vi "Begin.vi"(8 "error in":errorcluster) -> (0 "error out":errorcluster)   [LabVIEW 2017]
doc: "Called before other user functions, this VI is expected to open initial I/O refnums, load in file data, and do all program initialization. Notice that the <B>error out</B> terminal is simply used for data flow. Wiring it to other structures or subVIs ensures that this VI runs first."
uses:
  <vilib>/Rock Robotics/WPI/DriverStation/WPI_DriverStationRobotMode2.ctl
  <vilib>/Rock Robotics/WPI/Joystick/WPI_JoystickDeviceEnum.ctl
  <vilib>/Rock Robotics/SystemInterfaces/DIO/FPGA_DIOPWMChannel.ctl
  <vilib>/Rock Robotics/WPI/SafetyOutput/WPI_SafetyOutputConfigMenu.ctl
  Robot Global Data.vi
  <vilib>/Rock Robotics/Network Tables/NT Write String Array.vi
  <vilib>/Rock Robotics/WPI/MotorControl/WPI_MotorControlOpen VictorSP.vi
  <vilib>/Rock Robotics/WPI/MotorControl/WPI_MotorControlOpen SPARK.vi
  <vilib>/Rock Robotics/WPI/RobotDrive/WPI_RobotDriveOpen4MotorWithExistingMotors.vi
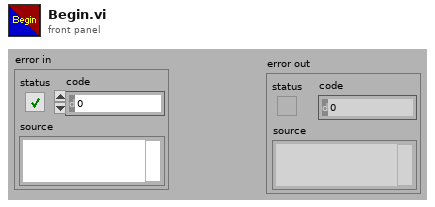
[diagram p1: front panel]
types:
  T1 = typedef "WPI_SafetyOutputConfigMenu.ctl" = enum16{"Enable", "Disable"}
  T2 = typedef "FPGA_DIOPWMChannel.ctl" = enum8{"PWM 0", "PWM 1", "PWM 2", "PWM 3", "PWM 4", "PWM 5", "PWM 6", "PWM 7", "PWM 8", "PWM 9", "PWM MXP 0", "PWM MXP 1", "PWM MXP 2", "PWM MXP 3", "PWM MXP 4", "PWM MXP 5", "PWM MXP 6", "PWM MXP 7", "PWM MXP 8", "PWM MXP 9", "Invalid"}
  T3 = typedef "WPI_JoystickDeviceEnum.ctl" = enum16{"USB 0", "USB 1", "USB 2", "USB 3", "USB 4", "USB 5"}
  T4 = typedef "WPI_DriverStationRobotMode2.ctl" = enum16{"Autonomous Disabled", "Autonomous Enabled", "Teleop Disabled", "Teleop Enabled", "Disconnected", "Finish", "Test Disabled", "Test Enabled", "Emergency Stopped"}
  T5 = typedef "WPI_JoystickDevRef.ctl" = cluster{"Device":T3}
  T6 = typedef "WPI_MotorControlDeviceRef.ctl" = cluster{"DeviceStatus":errorcluster, "Type":T7, "PWM":cluster{"PWM Channel":T2, "DeadBand":T8}, "CAN":cluster{"Device Number":u8, "SetOutput VI Ref":variant, "GetOutput VI Ref":variant, "Enable VI Ref":variant, "Disable VI Ref":variant, "Data":variant}, "Invert":bool, "DIO PWM":cluster{"PWM \"Enable\" Channel":T2, "DIOChannel":T9, "PWM Rate":dbl}}
  T7 = typedef "WPI_MotorControlType.ctl" = enum16{"PWM", "CAN", "DIO PWM"}
  T8 = typedef "WPI_PWMDeadband.ctl" = cluster{"Name":string, "maxPositivePwm":i32, "minPositivePwm":i32, "centerPwm":i32, "maxNegativePwm":i32, "minNegativePwm":i32, "angularRange":u16}
  T9 = typedef "FPGA_DIOChannel.ctl" = enum8{"DIO 0", "DIO 1", "DIO 2", "DIO 3", "DIO 4", "DIO 5", "DIO 6", "DIO 7", "DIO 8", "DIO 9", "DIO MXP 0", "DIO MXP 1", "DIO MXP 2", "DIO MXP 3", "DIO MXP 4", "DIO MXP 5", "DIO MXP 6", "DIO MXP 7", "DIO MXP 8", "DIO MXP 9", "DIO MXP 10", "DIO MXP 11", "DIO MXP 12", "DIO MXP 13", "DIO MXP 14", "DIO MXP 15", "SPI Port CS1", "SPI Port CS2", "SPI Port CS3", "SPI Port MISO", "SPI Port MOSI", "Invalid"}
  T10 = typedef "WPI_RobotDriveDevRef.ctl" = cluster{"DevStatus":errorcluster, "Motors[]":T6[], "Square Inputs":bool, "Max Output":dbl}
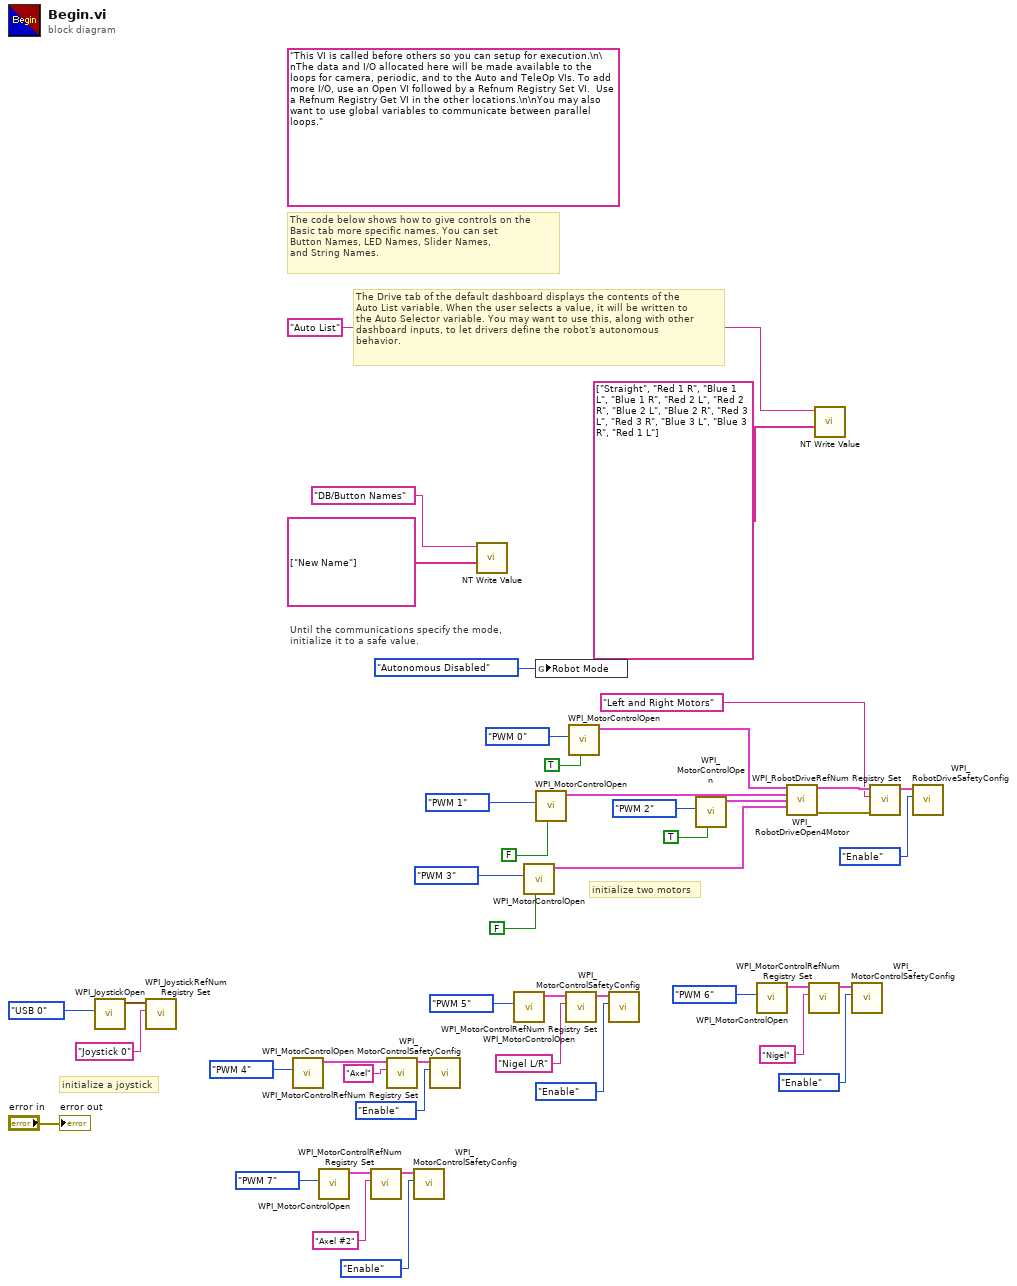
[diagram p0: block diagram]
diagram:
  (unwired) "This VI is called before others so you can setup for execution.\n\nThe data and I/O allocated here will be made available to the loops for camera, periodic, and to the Auto and TeleOp VIs. To add more I/O, use an Open VI followed by a Refnum Registry Set VI.  Use a Refnum Registry Get VI in the other locations.\n\nYou may also want to use global variables to communicate between parallel loops."
  # "The Drive tab of the default dashboard displays the contents of the\nAuto List variable. When the user selects a value, it will be written to\nthe Auto Selector variable. You may want to use this, along with other\ndashboard inputs, to let drivers define the robot's autonomous\nbehavior."
  # "The code below shows how to give controls on the\nBasic tab more specific names. You can set\nButton Names, LED Names, Slider Names,\nand String Names."
  # "initialize a joystick"
  # "Until the communications specify the mode,\ninitialize it to a safe value."
  # "initialize two motors"
  n1 = call <vilib>:"WPI_JoystickOpen.vi"("JoystickDevice"=WPI_JoystickDeviceEnum."USB 0") -> ("JoystickDevRef"=w39:T5)  [unwired: 10 in]
  n2 = call <vilib>:"WPI_JoystickRefNum Registry Set.vi"("refnum name"="Joystick 0", "JoystickDevRef"=w39) -> ()  [unwired: 8 in, 2 out]
  n3 = call-poly <vilib>:"WPI_MotorControlOpen.vi"("PWM Channel"=FPGA_DIOPWMChannel."PWM 4") -> ("MotorControlDeviceRef"=w23:T6)  [unwired: 9 in, 1 out]
  n4 = call-poly <vilib>:"WPI_MotorControlOpen.vi"("PWM Channel"=FPGA_DIOPWMChannel."PWM 7") -> ("MotorControlDeviceRef"=w17:T6)  [unwired: 9 in, 1 out]
  n5 = call <vilib>:"WPI_MotorControlRefNum Registry Set.vi"("refnum name"="Axel #2", "MotorControlDevRef"=w17) -> ("MotorControlDevRef"=w16:T6)  [unwired: 8 in, 1 out]
  n6 = call <vilib>:"WPI_MotorControlRefNum Registry Set.vi"("refnum name"="Axel", "MotorControlDevRef"=w23) -> ("MotorControlDevRef"=w21:T6)  [unwired: 8 in, 1 out]
  n7 = call <vilib>:"WPI_MotorControlSafetyConfig.vi"("mode"=WPI_SafetyOutputConfigMenu."Enable", "MotorControlDevRef"=w16) -> ()  [unwired: 8 in, 2 out]
  n8 = call <vilib>:"WPI_MotorControlSafetyConfig.vi"("mode"=WPI_SafetyOutputConfigMenu."Enable", "MotorControlDevRef"=w21) -> ()  [unwired: 8 in, 2 out]
  n9 = call-poly <vilib>:"NT Write Value.vi"("String Array"=string[] ["New Name"], "Name"="DB/Button Names") -> ()  [unwired: 9 in, 1 out]
  n10 = call-poly <vilib>:"WPI_MotorControlOpen.vi"("PWM Channel"=FPGA_DIOPWMChannel."PWM 5") -> ("MotorControlDeviceRef"=w11:T6)  [unwired: 9 in, 1 out]
  n11 = call-poly <vilib>:"WPI_MotorControlOpen.vi"("Invert"=FALSE, "PWM Channel"=FPGA_DIOPWMChannel."PWM 3") -> ("MotorControlDeviceRef"=w31:T6)  [unwired: 8 in, 1 out]
  n12 = global write "Robot Global Data.vi" "Robot Mode"(WPI_DriverStationRobotMode2."Autonomous Disabled" ("Robot Mode")) -> ()
  n13 = call-poly <vilib>:"WPI_MotorControlOpen.vi"("Invert"=FALSE, "PWM Channel"=FPGA_DIOPWMChannel."PWM 1") -> ("MotorControlDeviceRef"=w25:T6)  [unwired: 8 in, 1 out]
  n14 = call <vilib>:"WPI_MotorControlRefNum Registry Set.vi"("refnum name"="Nigel L/R", "MotorControlDevRef"=w11) -> ("MotorControlDevRef"=w9:T6)  [unwired: 8 in, 1 out]
  n15 = call-poly <vilib>:"WPI_MotorControlOpen.vi"("Invert"=TRUE, "PWM Channel"=FPGA_DIOPWMChannel."PWM 0") -> ("MotorControlDeviceRef"=w32:T6)  [unwired: 8 in, 1 out]
  n16 = call <vilib>:"WPI_MotorControlSafetyConfig.vi"("mode"=WPI_SafetyOutputConfigMenu."Enable", "MotorControlDevRef"=w9) -> ()  [unwired: 8 in, 2 out]
  n17 = call-poly <vilib>:"WPI_MotorControlOpen.vi"("Invert"=TRUE, "PWM Channel"=FPGA_DIOPWMChannel."PWM 2") -> ("MotorControlDeviceRef"=w30:T6)  [unwired: 8 in, 1 out]
  n18 = call-poly <vilib>:"WPI_MotorControlOpen.vi"("PWM Channel"=FPGA_DIOPWMChannel."PWM 6") -> ("MotorControlDeviceRef"=w6:T6)  [unwired: 9 in, 1 out]
  n19 = call-poly <vilib>:"WPI_RobotDriveOpen4Motor.vi"("Rear Left Motor Dev Ref"=w32, "Rear Right Motor Dev Ref"=w25, "Front Left Motor Dev Ref"=w30, "Front Right Motor Dev Ref"=w31) -> ("RobotDriveDevRef"=w46:T10, "error out"=w44:errorcluster)  [unwired: 10 in]
  n20 = call <vilib>:"WPI_MotorControlRefNum Registry Set.vi"("refnum name"="Nigel", "MotorControlDevRef"=w6) -> ("MotorControlDevRef"=w4:T6)  [unwired: 8 in, 1 out]
  n21 = call-poly <vilib>:"NT Write Value.vi"("String Array"=string[] ["Straight", "Red 1 R", "Blue 1 L", "Blue 1 R", "Red 2 L", "Red 2 R", "Blue 2 L", "Blue 2 R", "Red 3 L", "Red 3 R", "Blue 3 L", "Blue 3 R", "Red 1 L"], "Name"="Auto List") -> ()  [unwired: 9 in, 1 out]
  n22 = call <vilib>:"WPI_MotorControlSafetyConfig.vi"("mode"=WPI_SafetyOutputConfigMenu."Enable", "MotorControlDevRef"=w4) -> ()  [unwired: 8 in, 2 out]
  n23 = call <vilib>:"WPI_RobotDriveRefNum Registry Set.vi"("error in (no error)"=w44, "refnum name"="Left and Right Motors", "RobotDriveDevRef"=w46) -> ("RobotDriveDevRef"=w43:T10)  [unwired: 1 in, 7 out]
  n24 = call <vilib>:"WPI_RobotDriveSafetyConfig.vi"("mode"=WPI_SafetyOutputConfigMenu."Enable", "RobotDriveDevRef"=w43) -> ()  [unwired: 8 in, 2 out]
  "error out" <- "error in"
